vi "Create Event.vi"(9 "Event jettl":refnum<class "Event.lvclass">, 10 "Alias":string, 11 "Hello World Queue in":refnum<class "Hello World Queue.lvclass">) -> (3 "Hello World Queue out":refnum<class "Hello World Queue.lvclass">)   [LabVIEW 2021, in "Hello World Queue.lvlib" / "Hello World Queue.lvclass"]
uses:
  Hello World Queue.lvclass
  jettl/Event/Event.lvclass
  Hello World Queue.lvclass/Hello World Queue.ctl
  jettl/Queue/Queue.lvclass
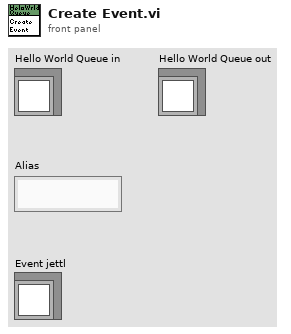
[diagram p1: front panel]
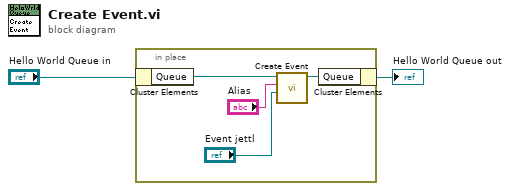
[diagram p0: block diagram]
diagram:
  n1 = in-place {
    n2 = in-place-cluster #1("Hello World Queue in") -> ("Queue"=w6:refnum<class "Queue.lvclass">)
    n3 = call-dynamic "Create Event.vi"("Event"="Event jettl", "Self Event Alias"="Alias", "Create Event in"=w6) -> ("Create Event out"=w5:refnum<class "Queue.lvclass">)  [unwired: 8 in]
    n4 = in-place-cluster #1("Queue"=w5) -> (→"Hello World Queue out":refnum<class "Hello World Queue.lvclass">)
  }
